vi "TCP Settings Dialog.vi"(11 "Message Queues out":T1) -> (3 "TCP Settings Out":cluster{"address":string, "port":u16})   [LabVIEW 2018, in "TCP Library.lvlib"]
uses:
  Lauda Integral XT-150 TCU/TCP Library.lvlib
  TCP Connection Settings.ctl
  Main/Main Queue Cluster.ctl
  support/Message Queue/Message Cluster.ctl
  support/Message Queue/Enqueue Message (Single).vi
  support/Message Queue/Message Queue.lvlib
panel:
  in  "error in (no error)":errorcluster
  out "error out":errorcluster
  out "OK":bool
  in  "Test":bool
  in  "TCP Settings In":T2={"address"="10.131.72.83", "port"=50023}
  in  "Cancel Button":bool
  in  "OK Button":bool
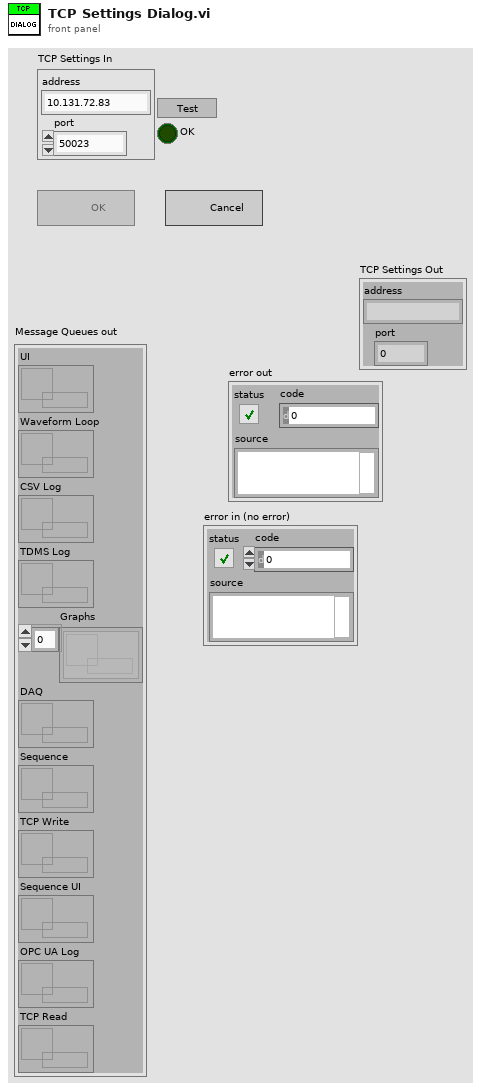
[diagram p1: front panel]
types:
  T1 = typedef "Main Queue Cluster.ctl" = cluster{"UI":refnum<queue>, "Waveform Loop":refnum<queue>, "CSV Log":refnum<queue>, "TDMS Log":refnum<queue>, "Graphs":refnum<queue>[], "DAQ":refnum<queue>, "Sequence":refnum<queue>, "TCP Write":refnum<queue>, "Sequence UI":refnum<queue>, "OPC UA Log":refnum<queue>, "TCP Read":refnum<queue>}
  T2 = typedef "TCP Library.lvlib/TCP Connection Settings.ctl" = cluster{"address":string, "port":u16}
  T3 = enum8{"Enabled", "Disabled", "Disabled and Grayed Out"}
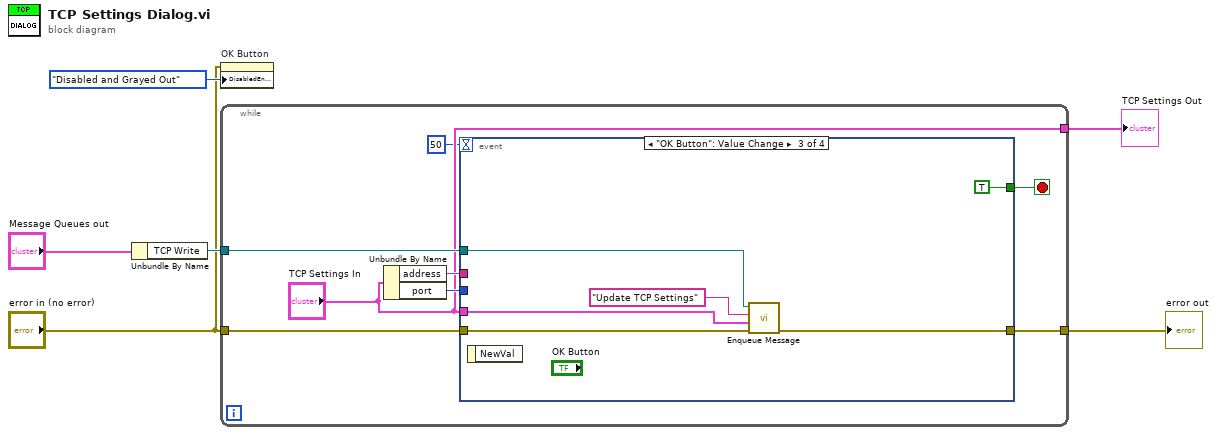
[diagram p0: block diagram]
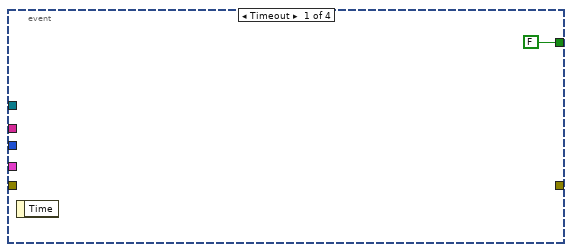
[diagram p2: hidden frame]
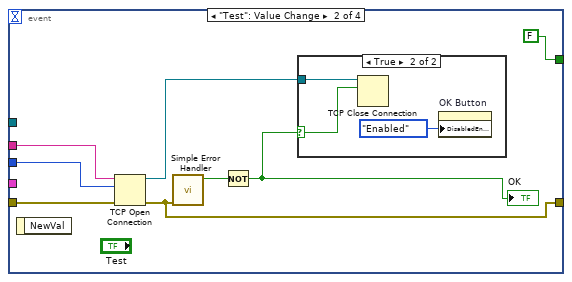
[diagram p3: hidden frame]
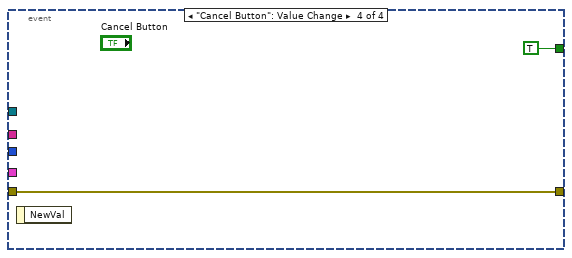
[diagram p5: hidden frame]
diagram:
  n1 = Unbundle By Name("Message Queues out") -> ("TCP Write"=w4:refnum<queue>)
  n2 = property on="OK Button" class="Bool"(error in="error in (no error)", "DisabledEnum"=T3."Disabled and Grayed Out" ("Disabled")) -> ()  [unwired: 1 in, 2 out]
  n3 = while {
    tunnel: "error in (no error)" -> [w14]
    tunnel: [w13] -> w6
    tunnel: w4 -> [w11]
    tunnel: ["TCP Settings In"] -> w1
    stop <- w12 stop-if-true
    n4 = Unbundle By Name("TCP Settings In") -> ("address"=w10:string, "port"=w9:u16)
    n5 = event shown="[2] \"OK Button\": Value Change" {
      selector: _ -> [_ _ _ _]
      dyn-events: _ -> [_ _ _ _]
      timeout: 50 -> [_ _ _ _]
      tunnel: w10 -> [_ w23 _ _]
      tunnel: w9 -> [_ w22 _ _]
      tunnel: [_ w20 w27 w33] -> w13
      tunnel: w14 -> [_ w21 w30 w33]
      tunnel: [FALSE FALSE TRUE TRUE] -> w12
      tunnel: w11 -> [_ _ w31 _]
      tunnel: "TCP Settings In" -> [_ _ w29 _]
      event Timeout {
        n6 = event-data() -> ()  [unwired: 1 in, 1 out]
      }
      event "Test": Value Change {
        n7 = event-data() -> ()  [unwired: 1 in, 1 out]
        n8 = TCP Open Connection(address=w23, remote port or service name=w22, error in (no error)=w21) -> (connection ID=w17:refnum<k5>, error out=w20:errorcluster)  [unwired: 2 in]
        n9 = call <vilib>:"Simple Error Handler.vi"("error in (no error)"=w20) -> ("error?"=w19:bool)  [unwired: 4 in, 4 out]
        n10 = Not(x=w19) -> (.not. x?=w18:bool)
        "OK" <- w18
        n11 = case shown="True" w18 {
          selector: w18 -> [_ w26]
          tunnel: w17 -> [_ w25]
          frame False {
          }
          frame True {
            n12 = TCP Close Connection(connection ID=w25, abort (F)=w26) -> ()  [unwired: 1 in, 2 out]
            n13 = property on="OK Button" class="Bool"("DisabledEnum"=T3."Enabled" ("Disabled")) -> ()  [unwired: 2 in, 2 out]
          }
        }
      }
      event "OK Button": Value Change {
        n14 = event-data() -> ()  [unwired: 1 in, 1 out]
        n15 = call-poly "Enqueue Message.vi"("error in (no error)"=w30, "Message Data"=w29, "Message"="Update TCP Settings", "Message Queue"=w31) -> ("error out"=w27:errorcluster)  [unwired: 6 in, 1 out]
      }
      event "Cancel Button": Value Change {
        n16 = event-data() -> ()  [unwired: 1 in, 1 out]
      }
    }
  }
  "error out" <- w6
  "TCP Settings Out" <- w1
